vi "converterPartNumber.vi"(11 "bytes [0, 1, 2]":string) -> (3 "PartNumber":string)   [LabVIEW 2018]
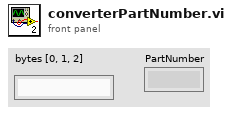
[diagram p1: front panel]
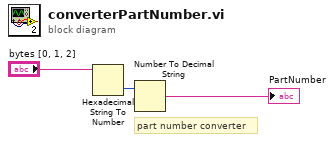
[diagram p0: block diagram]
diagram:
  # "part number converter"
  n1 = Hexadecimal String To Number(string="bytes [0, 1, 2]") -> (number=w2:u32)  [unwired: 2 in, 1 out]
  n2 = Number To Decimal String(number=w2) -> (decimal integer string=→"PartNumber":string)  [unwired: 1 in]
